vi "CAD@MotionTable__Parameter.vi"(1 "ParamterIn":string) -> (0 "ParamterOut":string)   [LabVIEW 2019]
panel:
  in  "Action":string(combo)
  in  "Confirm":bool
  # "CAD@MotionTable $Action"
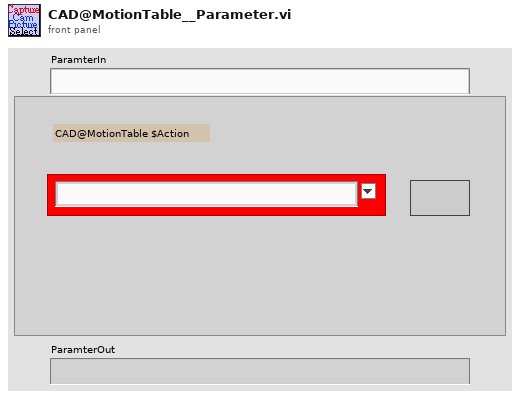
[diagram p1: front panel]
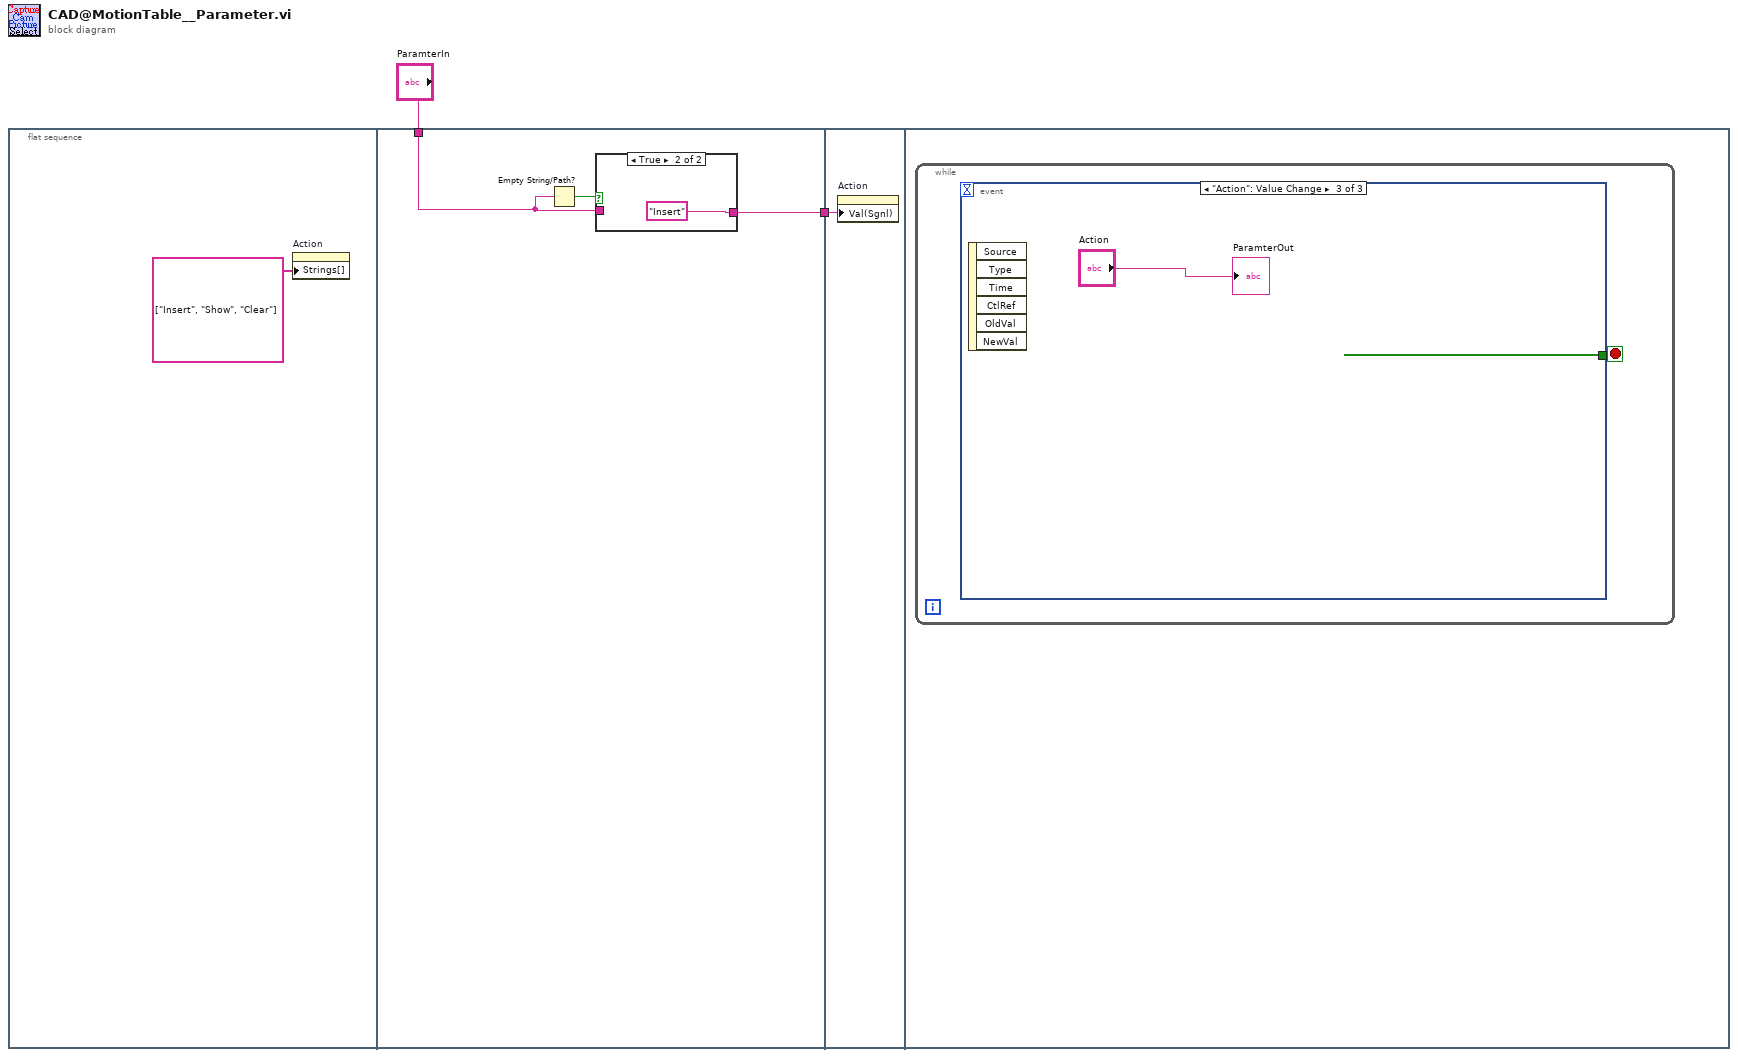
[diagram p0: block diagram]
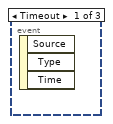
[diagram p3: hidden frame]
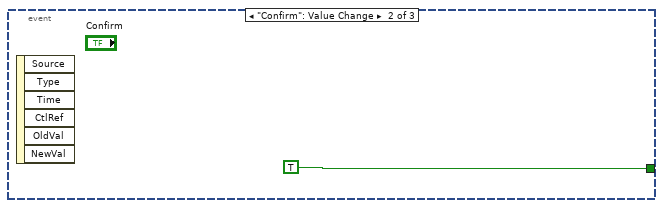
[diagram p4: hidden frame]
diagram:
  n1 = flat-sequence {
    tunnel: "ParamterIn" -> [w4]
    tunnel: [w5] -> w1
    tunnel: w1 -> [w9]
    frame #0 {
      n2 = property on="Action" class="CmbBox"("Strings[]"=string[] ["Insert", "Show", "Clear"] ("Strings []")) -> ()  [unwired: 2 in, 2 out]
    }
    frame #1 {
      n3 = Empty String/Path?(string/path=w4) -> (empty?=w6:bool)
      n4 = case shown="True" w6 {
        tunnel: w4 -> [w7 _]
        tunnel: [w7 "Insert"] -> w5
        frame False {
        }
        frame True {
        }
      }
    }
    frame #2 {
      n5 = property on="Action" class="CmbBox"("Val(Sgnl)"=w9) -> ()  [unwired: 2 in, 2 out]
    }
    frame #3 {
      n6 = while {
        stop <- w10 stop-if-true
        n7 = event shown="[2] \"Action\": Value Change" {
          selector: _ -> [_ _ _]
          dyn-events: _ -> [_ _ _]
          timeout: _ -> [_ _ _]
          tunnel: [_ TRUE _] -> w10
          event Timeout {
            n8 = event-data() -> ()  [unwired: 1 in, 3 out]
          }
          event "Confirm": Value Change {
            n9 = event-data() -> ()  [unwired: 1 in, 6 out]
          }
          event "Action": Value Change {
            n10 = event-data() -> ()  [unwired: 1 in, 6 out]
            "ParamterOut" <- "Action"
          }
        }
      }
    }
  }
